vi "Configure Port Extension Characteristics.vi"(0 "VISA resource name":refnum<visa-resource-name>, 1 "Enable Loss and Frequency (F: Disable)":bool, 2 "DC Loss Value (0)":dbl, 5 "Channel (1)":i32=1, 7 "Port (1)":i32=1, 9 "Include Number (1)":i32=1, 11 "error in (no error)":errorcluster, 12 "Loss Value (0 dB)":dbl, 13 "Frequency Value (1E+9)":dbl=1000000000.0) -> (4 "VISA resource name out":refnum<visa-resource-name>, 15 "error out":errorcluster)   [LabVIEW 2020, in "Agilent ENA Series.lvlib"]
doc: "Configures the port extension characteristic settings.\n\n<B>Note:</B>\nThis VI is only valid for E5061B, E5070B and E5071B."
uses:
  <instrlib>/Agilent ENA Series/Agilent ENA Series.lvlib
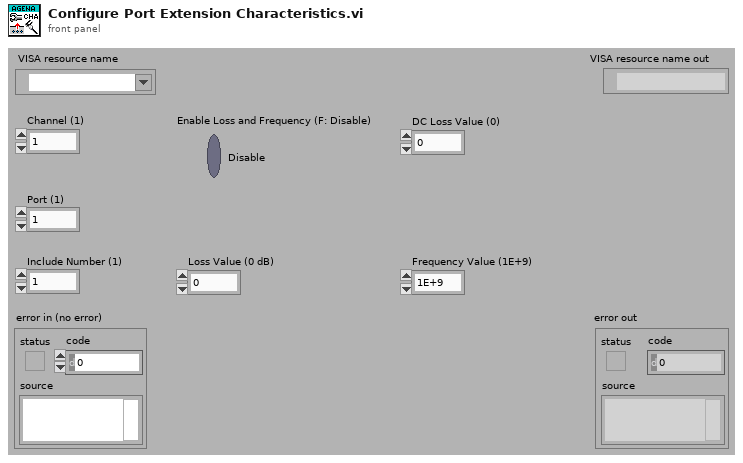
[diagram p1: front panel]
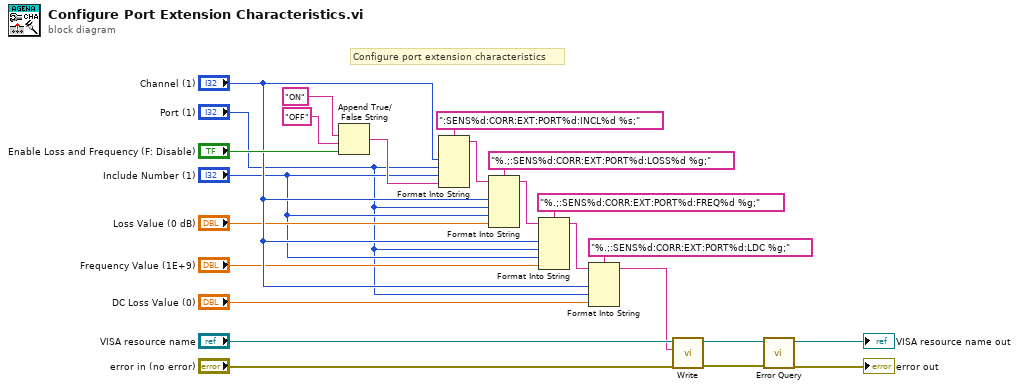
[diagram p0: block diagram]
diagram:
  # "Configure port extension characteristics"
  n1 = Append True/False String(1:"Enable Loss and Frequency (F: Disable)", 2:"OFF", 3:"ON") -> (0:w19:string)  [unwired: 1 out]
  n2 = Format Into String(format string=":SENS%d:CORR:EXT:PORT%d:INCL%d %s;", "Channel (1)", "Port (1)", "Include Number (1)", w19) -> (resulting string=w18:string)  [unwired: 2 in, 1 out]
  n3 = Format Into String(format string="%.;:SENS%d:CORR:EXT:PORT%d:LOSS%d %g;", initial string=w18, "Channel (1)", "Port (1)", "Include Number (1)", "Loss Value (0 dB)") -> (resulting string=w15:string)  [unwired: 1 in, 1 out]
  n4 = Format Into String(format string="%.;:SENS%d:CORR:EXT:PORT%d:FREQ%d %g;", initial string=w15, "Channel (1)", "Port (1)", "Include Number (1)", "Frequency Value (1E+9)") -> (resulting string=w12:string)  [unwired: 1 in, 1 out]
  n5 = Format Into String(format string="%.;:SENS%d:CORR:EXT:PORT%d:LDC %g;", initial string=w12, "Channel (1)", "Port (1)", "DC Loss Value (0)") -> (resulting string=w1:string)  [unwired: 1 in, 1 out]
  n6 = call <instrlib>:"Write.vi"("error in (no error)"="error in (no error)", "String ()"=w1, "VISA resource name"="VISA resource name") -> ("error out"=w4:errorcluster, "VISA resource name out"=w5:refnum<visa-resource-name>)  [unwired: 6 in, 1 out]
  n7 = call <instrlib>:"Error Query.vi"("error in (no error)"=w4, "VISA resource name"=w5) -> ("error out"=→"error out":errorcluster, "VISA resource name out"=→"VISA resource name out":refnum<visa-resource-name>)  [unwired: 8 out]
